vi "Set Initialization Data - Acquire.vi"(8 "error in":errorcluster, 11 "Manager Worker in":refnum<class "Manager Worker.lvclass">) -> (0 "error out":errorcluster, 3 "Manager Worker out":refnum<class "Manager Worker.lvclass">)   [LabVIEW 2018, in "Manager Worker.lvclass"]
doc: "Sets the initialization data of a statically linked subWorker."
uses:
  Manager Worker.lvclass
  D:/Program Files (x86)/National Instruments/LabVIEW 2018/vi.lib/addons/_Workers/Library/Classes/Worker/Worker.lvclass
  Acquire Worker/Initialization Data.ctl
  <vilib>/addons/_Workers/Library/Classes/Message Queue/Message Queue.lvclass
  <vilib>/addons/_Workers/Library/Classes/Worker/Worker.lvclass/Worker.ctl
  Manager Worker.lvclass/Manager Worker.ctl
  ChartView Worker/ChartView Worker.lvclass
  Acquire Worker/DataAcquire Worker.lvclass
  <vilib>/addons/_Workers/Library/Classes/Worker/Worker.lvclass
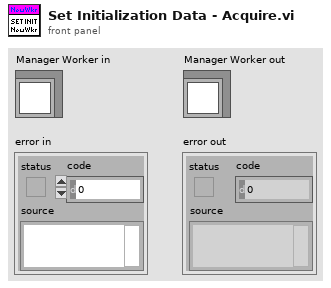
[diagram p1: front panel]
types:
  T1 = typedef "DataAcquire Worker.lvclass/Initialization Data.ctl" = cluster{"String":string, "Manager Queue":refnum<class "Message Queue.lvclass">, "Chart Queue":refnum<class "Message Queue.lvclass">}
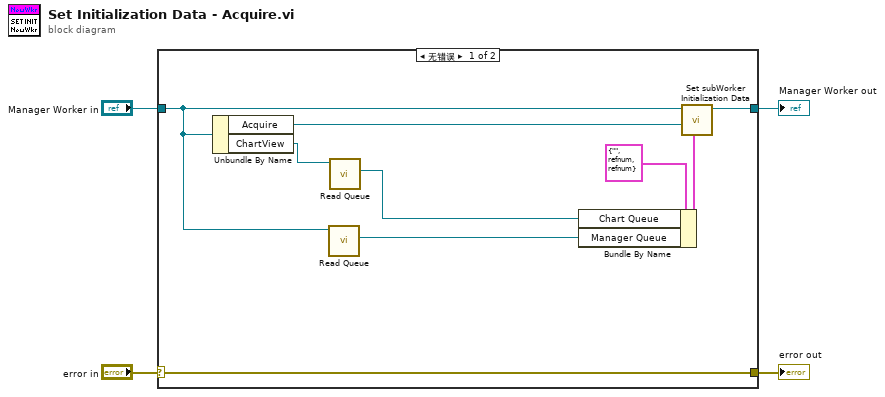
[diagram p0: block diagram]
diagram:
  n1 = case shown="无错误" "error in" {
    selector: "error in" -> [w13 w15]
    tunnel: [w13 w15] -> w3
    tunnel: [w11 w14] -> w2
    tunnel: "Manager Worker in" -> [w8 w14]
    frame No Error {
      n2 = Unbundle By Name(w8) -> ("Acquire"=w12:refnum<class "DataAcquire Worker.lvclass">, "ChartView"=w6:refnum<class "ChartView Worker.lvclass">)
      n3 = call <vilib>:"Read Queue.vi"("Worker"=w8) -> ("Message Queue out"=w7:refnum<class "Message Queue.lvclass">)  [unwired: 9 in, 1 out]
      n4 = call <vilib>:"Read Queue.vi"("Worker"=w6) -> ("Message Queue out"=w5:refnum<class "Message Queue.lvclass">)  [unwired: 9 in, 1 out]
      n5 = Bundle By Name(cluster=T1 {"String"="", "Manager Queue"=refnum, "Chart Queue"=refnum} ("Initialization Data"), "Chart Queue"=w5, "Manager Queue"=w7) -> (w9:T1)
      n6 = call-dynamic "Set subWorker Initialization Data.vi"("Initialization Data"=w9, "subWorker"=w12, "Worker"=w8) -> ("Worker out"=w11:refnum<class "Manager Worker.lvclass">)  [unwired: 8 in]
    }
    frame Error {
    }
  }
  "error out" <- w3
  "Manager Worker out" <- w2
